vi "morztolett.vi"(1 "String":string) -> (0 "String 2":string)   [LabVIEW 2015]
panel:
  in  "Array 2":string[](array[string])
  in  "Array":string[](array[string])
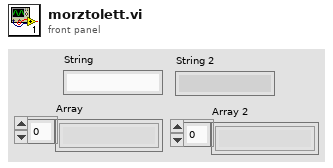
[diagram p1: front panel]
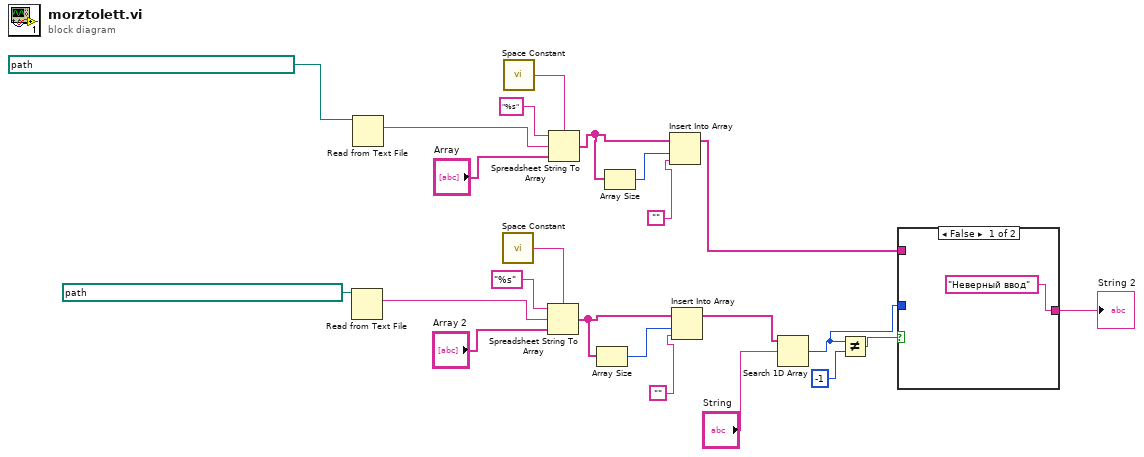
[diagram p0: block diagram]
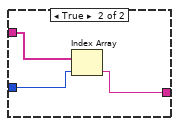
[diagram p2: hidden frame]
diagram:
  n1 = Read from Text File(file (use dialog)=path "C:/Users/Валерия/Desktop/Новая папка/morz.txt") -> (text=w19:string)  [unwired: 3 in, 3 out]
  n2 = Read from Text File(file (use dialog)=path "C:/Users/Валерия/Desktop/Новая папка/alf.txt") -> (text=w23:string)  [unwired: 3 in, 3 out]
  n3 = call <vilib>:"Space Constant.vi"() -> ("String"=w18:string)
  n4 = call <vilib>:"Space Constant.vi"() -> ("String"=w22:string)
  n5 = Spreadsheet String To Array(delimiter (Tab)=w18, format string="%s", spreadsheet string=w19, array type (2D Dbl)="Array 2") -> (array=w14:string[])
  n6 = Spreadsheet String To Array(delimiter (Tab)=w22, format string="%s", spreadsheet string=w23, array type (2D Dbl)="Array") -> (array=w3:string[])
  n7 = Array Size(array=w14) -> (size(s)=w13:i32)
  n8 = Array Size(array=w3) -> (size(s)=w10:i32)
  n9 = Insert Into Array(array=w3, index=w10, new element="") -> (w5:string[])
  n10 = Insert Into Array(array=w14, index=w13, new element="") -> (w11:string[])
  n11 = Search 1D Array(1D array=w11, element="String") -> (index of element=w6:i32)  [unwired: 1 in]
  n12 = Not Equal?(x=w6, y=-1) -> (x != y?=w8:bool)
  n13 = case shown="False" w8 {
    tunnel: w6 -> [_ w26]
    tunnel: w5 -> [_ w27]
    tunnel: ["Неверный ввод" w25] -> w4
    frame False {
    }
    frame True {
      n14 = Index Array(array=w27, index=w26) -> (element=w25:string)
    }
  }
  "String 2" <- w4
